vi "rfStateChange.vi"(8 "error in (no error)":errorcluster, 11 "StaticOutputEditor in":refnum<class "StaticOutputEditor.lvclass">) -> (0 "error out":errorcluster, 3 "StaticOutputEditor out":refnum<class "StaticOutputEditor.lvclass">)   [LabVIEW 2011, in "Views.lvlib" / "ScriptEditor.lvlib" / "StaticOutputEditor.lvclass"]
uses:
  StaticOutputEditor.lvclass
  StaticOutputEditor.lvclass/StaticOutputEditor.ctl
  Tools/DatabaseHelpers/Database Objects/ChannelArray/ChannelArray.lvclass
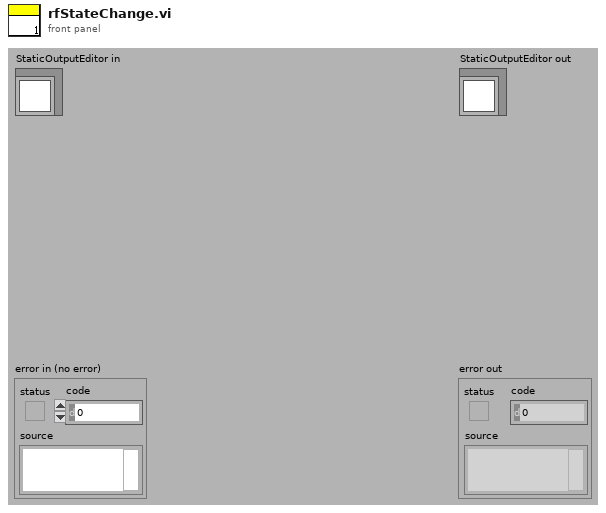
[diagram p1: front panel]
types:
  T1 = cluster{"state_name":string, "value":cluster{"frequency":string, "amplitude":string, "phase":string}}
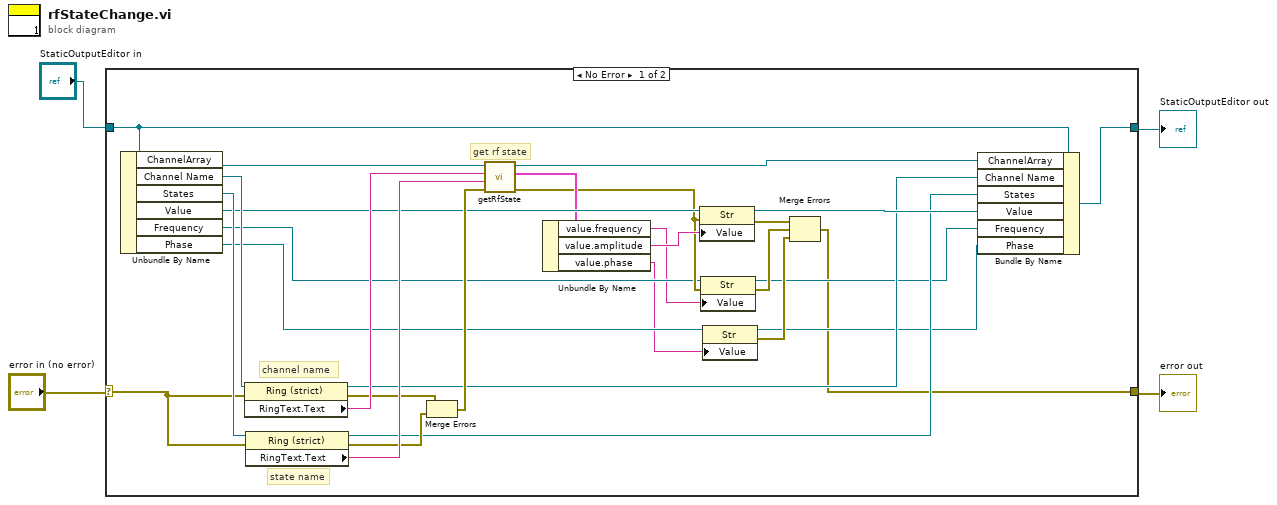
[diagram p0: block diagram]
diagram:
  n1 = case shown="No Error" "error in (no error)" {
    selector: "error in (no error)" -> [w28 w35]
    tunnel: [w5 w35] -> w3
    tunnel: [w6 w34] -> w1
    tunnel: "StaticOutputEditor in" -> [w9 w34]
    frame No Error {
      # "state name"
      # "channel name"
      # "get rf state"
      n2 = Unbundle By Name(w9) -> ("ChannelArray"=w32:refnum<class "ChannelArray.lvclass">, "Channel Name"=w31:refnum<vi>, "States"=w30:refnum<vi>, "Value"=w23:refnum<vi>, "Frequency"=w19:refnum<vi>, "Phase"=w17:refnum<vi>)
      n3 = property class="Ring (strict)"(reference=w31, error in=w28) -> (reference out=w11:refnum<vi>, error out=w26:errorcluster, "RingText.Text"=w27:string)
      n4 = property class="Ring (strict)"(reference=w30, error in=w28) -> (reference out=w10:refnum<vi>, error out=w25:errorcluster, "RingText.Text"=w29:string)
      n5 = Merge Errors(w26, w25) -> (w24:errorcluster)
      n6 = call "getRfState.vi"("error in (no error)"=w24, "state_name"=w29, "channel_name"=w27, "ChannelArray in"=w32) -> ("error out"=w20:errorcluster, "rf_state"=w22:T1, "ChannelArray out"=w12:refnum<class "ChannelArray.lvclass">)  [unwired: 5 in]
      n7 = Unbundle By Name(w22) -> ("value.frequency"=w18:string, "value.amplitude"=w21:string, "value.phase"=w16:string)
      n8 = property class="Str"(reference=w23, error in=w20, "Value"=w21) -> (reference out=w33:refnum<vi>, error out=w15:errorcluster)
      n9 = property class="Str"(reference=w19, error in=w20, "Value"=w18) -> (reference out=w8:refnum<vi>, error out=w14:errorcluster)
      n10 = property class="Str"(reference=w17, "Value"=w16) -> (reference out=w7:refnum<vi>, error out=w13:errorcluster)  [unwired: 1 in]
      n11 = Merge Errors(w15, w14, w13) -> (w5:errorcluster)
      n12 = Bundle By Name(cluster=w9, "ChannelArray"=w12, "Channel Name"=w11, "States"=w10, "Value"=w33, "Frequency"=w8, "Phase"=w7) -> (w6:refnum<class "StaticOutputEditor.lvclass">)
    }
    frame Error {
    }
  }
  "error out" <- w3
  "StaticOutputEditor out" <- w1
